vi "processCamera.vi"(0 "S arrays":T2, 1 "index":i32, 3 "B [T]":dbl=1.0, 5 "Clibration":T7={"cam 0"={"incident ANGLE COMPENSATION"=[], "field of view /pixel"=0.0, "dp/B [MeV/C/B]"=[], "charge compensation"=[], "Momentum [MeV/C]"=[], "B [T]"=1.0, "energyDependence Input"=[], "pixel angle (y)"=[], "dp [MeV/C/] "=[], "angle 2Dfor spectrumj"=[], "dp [MeV/C] 2D"=[], "charge compensation 2D"=[], "Screen&Camera 2"={"Screen Orientation"="Regular", "Screen angle"="Flat", "Lens"=enum."FL1-f8x08", "Calibration (mm/pix)"=1.0}, "ROI info"={"npix-X"=0, "npix-Y"=0, "Left [pix]"=0.0, "Top [pix]"=0.0}, "Y 2D full angle"=[]}, "cam 1"={"incident ANGLE COMPENSATION"=[], "field of view /pixel"=0.0, "dp/B [MeV/C/B]"=[], "charge compensation"=[], "Momentum [MeV/C]"=[], "B [T]"=1.0, "energyDependence Input"=[], "pixel angle (y)"=[], "dp [MeV/C/] "=[], "angle 2Dfor spectrumj"=[], "dp [MeV/C] 2D"=[], "charge compensation 2D"=[], "Screen&Camera 2"={"Screen Orientation"="Regular", "Screen angle"="Flat", "Lens"=enum."FL1-f8x08", "Calibration (mm/pix)"=1.0}, "ROI info"={"npix-X"=0, "npix-Y"=0, "Left [pix]"=0.0, "Top [pix]"=0.0}, "Y 2D full angle"=[]}, "cam 2"={"incident ANGLE COMPENSATION"=[], "field of view /pixel"=0.0, "dp/B [MeV/C/B]"=[], "charge compensation"=[], "Momentum [MeV/C]"=[], "B [T]"=1.0, "energyDependence Input"=[], "pixel angle (y)"=[], "dp [MeV/C/] "=[], "angle 2Dfor spectrumj"=[], "dp [MeV/C] 2D"=[], "charge compensation 2D"=[], "Screen&Camera 2"={"Screen Orientation"="Regular", "Screen angle"="Flat", "Lens"=enum."FL1-f8x08", "Calibration (mm/pix)"=1.0}, "ROI info"={"npix-X"=0, "npix-Y"=0, "Left [pix]"=0.0, "Top [pix]"=0.0}, "Y 2D full angle"=[]}, "cam 3"={"incident ANGLE COMPENSATION"=[], "field of view /pixel"=0.0, "dp/B [MeV/C/B]"=[], "charge compensation"=[], "Momentum [MeV/C]"=[], "B [T]"=1.0, "energyDependence Input"=[], "pixel angle (y)"=[], "dp [MeV/C/] "=[], "angle 2Dfor spectrumj"=[], "dp [MeV/C] 2D"=[], "charge compensation 2D"=[], "Screen&Camera 2"={"Screen Orientation"="Regular", "Screen angle"="Flat", "Lens"=enum."FL1-f8x08", "Calibration (mm/pix)"=1.0}, "ROI info"={"npix-X"=0, "npix-Y"=0, "Left [pix]"=0.0, "Top [pix]"=0.0}, "Y 2D full angle"=[]}}, 9 "CamSettings":T3={"Cam 0"={"position"=0.0, "Field of view"=0.0, "start"=0.0, "end"=0.0, "center"=0.0, "Lens"=enum."FL1-f8x08", "Forward"=enum."off", "Spec_Calib_file 2"=path "Y:/100TWdata/ESMCalib/datFwd.txt", "map"=path "Y:/100TWdata/ESMCalib/mapFwd.txt", "y size"=0}, "Cam 1"={"position"=0.0, "Field of view"=0.0, "start"=0.0, "end"=0.0, "center"=0.0, "Lens"=enum."FL1-f8x08", "Forward"=enum."off", "Spec_Calib_file 2"=path "Y:/100TWdata/ESMCalib/datFwd.txt", "map"=path "Y:/100TWdata/ESMCalib/mapFwd.txt", "y size"=0}, "Cam 2"={"position"=0.0, "Field of view"=0.0, "start"=0.0, "end"=0.0, "center"=0.0, "Lens"=enum."FL1-f8x08", "Forward"=enum."off", "Spec_Calib_file 2"=path "Y:/100TWdata/ESMCalib/datFwd.txt", "map"=path "Y:/100TWdata/ESMCalib/mapFwd.txt", "y size"=0}, "Cam 3"={"position"=0.0, "Field of view"=0.0, "start"=0.0, "end"=0.0, "center"=0.0, "Lens"=enum."FL1-f8x08", "Forward"=enum."off", "Spec_Calib_file 2"=path "Y:/100TWdata/ESMCalib/datFwd.txt", "map"=path "Y:/100TWdata/ESMCalib/mapFwd.txt", "y size"=0}}, 11 "error in (no error)":errorcluster, 12 "image in":T1, 14 "bg in":T1) -> (4 "z":dbl[][](graph), 6 "spec cluster":cluster{"dp [MeV/C]":dbl[], dbl[]}(graph), 8 "time: AllProc":u32, 10 "Cam Cluster out 2":T8={"incident ANGLE COMPENSATION"=[], "field of view /pixel"=0.0, "dp/B [MeV/C/B]"=[], "charge compensation"=[], "Momentum [MeV/C]"=[], "B [T]"=1.0, "energyDependence Input"=[], "pixel angle (y)"=[], "dp [MeV/C/] "=[], "angle 2Dfor spectrumj"=[], "dp [MeV/C] 2D"=[], "charge compensation 2D"=[], "Screen&Camera 2"={"Screen Orientation"="Regular", "Screen angle"="Flat", "Lens"=enum."FL1-f8x08", "Calibration (mm/pix)"=1.0}, "ROI info"={"npix-X"=0, "npix-Y"=0, "Left [pix]"=0.0, "Top [pix]"=0.0}, "Y 2D full angle"=[]}, 13 "Sum Y":cluster{"Ramp Pattern":dbl[], dbl[]}, 15 "error out":errorcluster)   [LabVIEW 2011, in "MagAnalysis_Online.lvclass"]
uses:
  MagAnalysis_Online.lvclass
  calib_Sub_Typdef.ctl
  ScreenCam2_TypDEf.ctl
  CamAndObj_TypDEf.ctl
  ROIInfo_TypDef.ctl
  Calib_Typdef.ctl
  CamSettings_Typdef.ctl
  CamSettingSUB_TypDEf.ctl
  OnOffTypeDef.ctl
  IMAQ Image.ctl
panel:
  out "time: cluster":u32
  out "time: process image":u32
  out "time:BG+Screws":u32
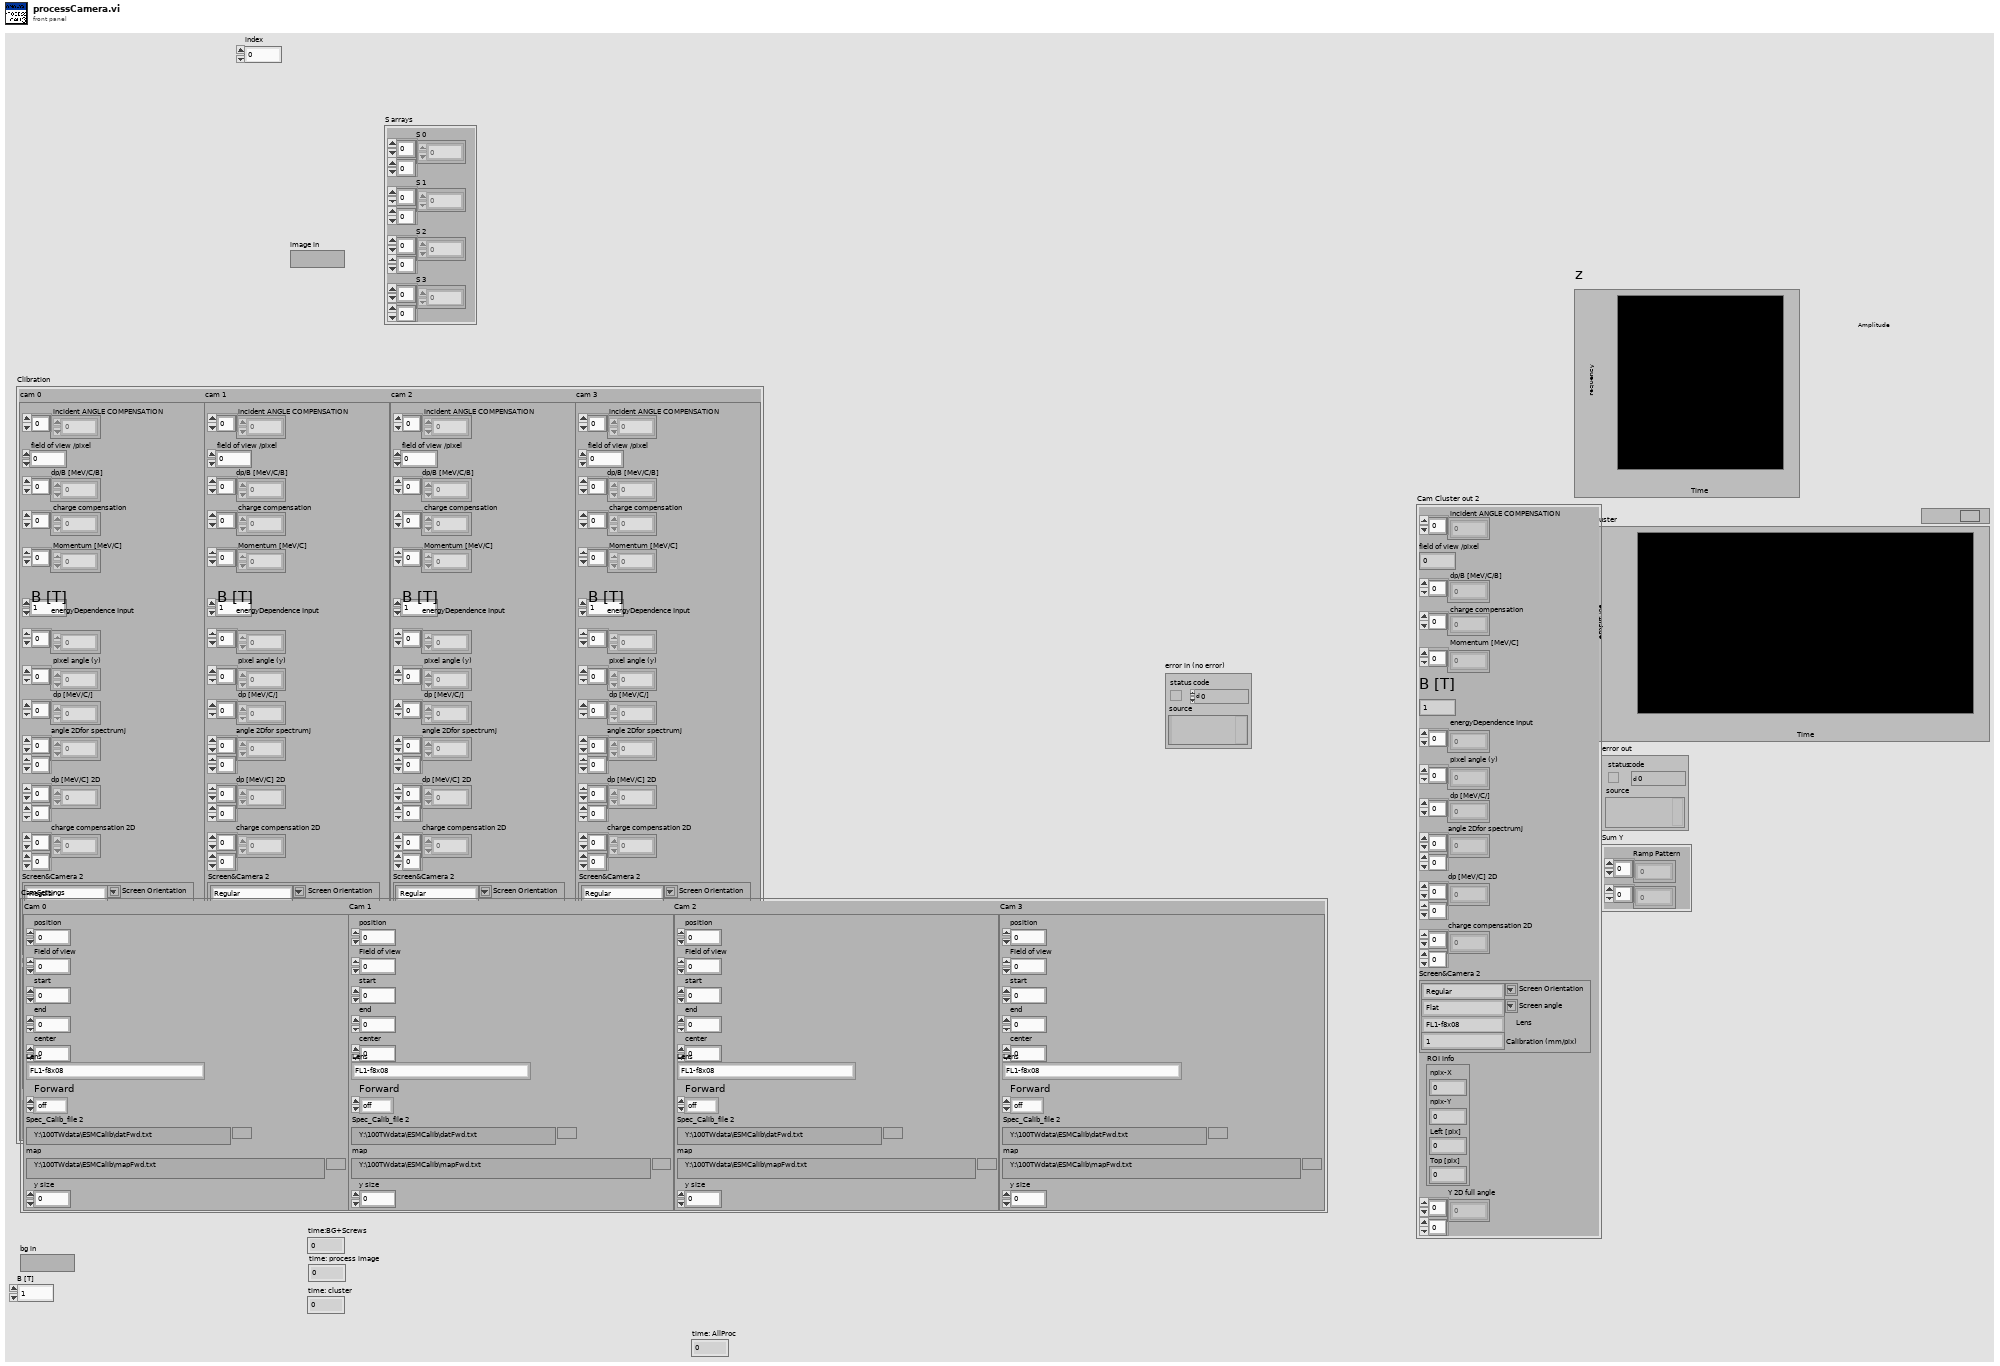
[diagram p1: front panel]
types:
  T1 = typedef "IMAQ Image.ctl" = refnum<image>
  T2 = cluster{"S 0":i32[][], "S 1":i32[][], "S 2":i32[][], "S 3":i32[][]}
  T3 = typedef "CamSettings_Typdef.ctl" = cluster{"Cam 0":T4, "Cam 1":T4, "Cam 2":T4, "Cam 3":T4}
  T4 = typedef "CamSettingSUB_TypDEf.ctl" = cluster{"position":dbl, "Field of view":dbl, "start":dbl, "end":dbl, "center":dbl, "Lens":T5, "Forward":T6, "Spec_Calib_file 2":path, "map":path, "y size":i32}
  T5 = typedef "CamAndObj_TypDEf.ctl" = enum16{"FL1-f8x08", "FL1-f8x06", "FL1-f8", "ch300-f50", "FL2G-f8", "FL3M14-f8", "FL3M14-f8x08", "FL3M14-f8x08(2x2)"}
  T6 = typedef "OnOffTypeDef.ctl" = enum16{"off", "on"}
  T7 = typedef "Calib_Typdef.ctl" = cluster{"cam 0":T8, "cam 1":T8, "cam 2":T8, "cam 3":T8}
  T8 = typedef "calib_Sub_Typdef.ctl" = cluster{"incident ANGLE COMPENSATION":dbl[], "field of view /pixel":dbl, "dp/B [MeV/C/B]":dbl[], "charge compensation":dbl[], "Momentum [MeV/C]":dbl[], "B [T]":dbl, "energyDependence Input":dbl[], "pixel angle (y)":dbl[], "dp [MeV/C/] ":dbl[], "angle 2Dfor spectrumj":dbl[][], "dp [MeV/C] 2D":dbl[][], "charge compensation 2D":dbl[][], "Screen&Camera 2":T9, "ROI info":T10, "Y 2D full angle":dbl[][]}
  T9 = typedef "ScreenCam2_TypDEf.ctl" = cluster{"Screen Orientation":string, "Screen angle":string, "Lens":T5, "Calibration (mm/pix)":dbl}
  T10 = typedef "ROIInfo_TypDef.ctl" = cluster{"npix-X":i32, "npix-Y":i32, "Left [pix]":dbl, "Top [pix]":dbl}
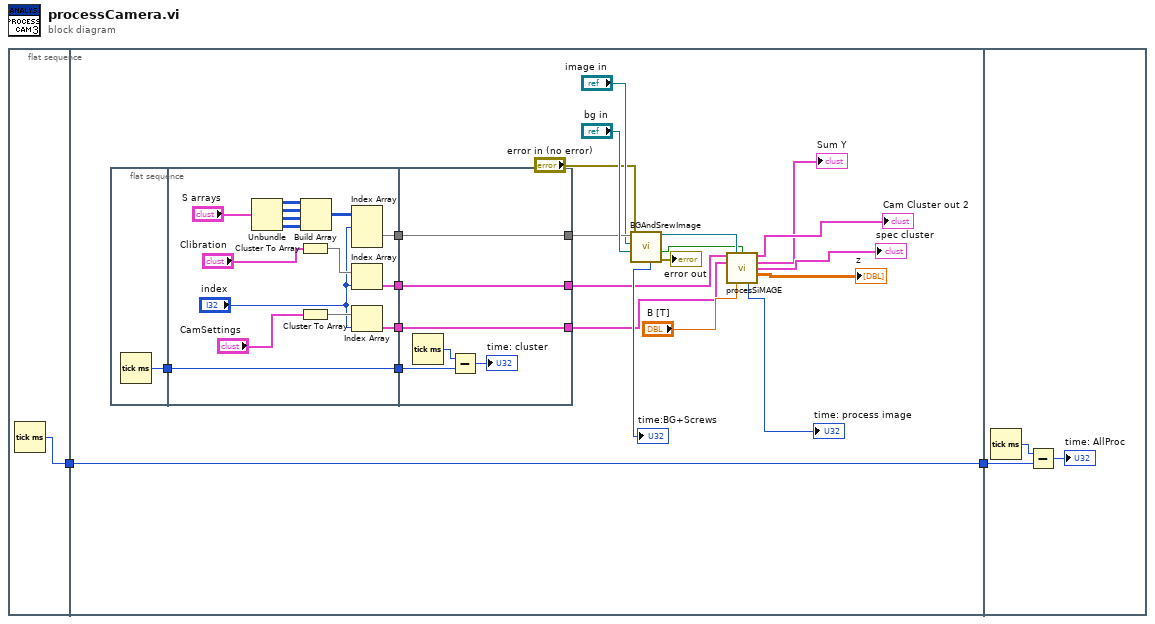
[diagram p0: block diagram]
diagram:
  n1 = flat-sequence {
    tunnel: [w3] -> w1
    tunnel: [w12] -> w2
    tunnel: w1 -> [w12]
    tunnel: w2 -> [w48]
    frame #0 {
      n2 = Tick Count (ms)() -> (millisecond timer value=w3:u32)
    }
    frame #1 {
      n3 = flat-sequence {
        tunnel: [w26] -> w25
        tunnel: [w38] -> w24
        tunnel: [w35] -> w23
        tunnel: [w27] -> w22
        tunnel: w25 -> [w41]
        tunnel: [w41] -> w21
        tunnel: [w45] -> w15
        tunnel: [w46] -> w13
        tunnel: [w47] -> w14
        tunnel: w24 -> [w47]
        tunnel: w23 -> [w46]
        tunnel: w22 -> [w45]
        tunnel: w21 -> [w42]
        frame #0 {
          n4 = Tick Count (ms)() -> (millisecond timer value=w26:u32)
        }
        frame #1 {
          n5 = Unbundle("S arrays") -> ("S 0"=w33:i32[][], "S 1"=w32:i32[][], "S 2"=w31:i32[][], "S 3"=w30:i32[][])
          n6 = Cluster To Array(cluster="Clibration") -> (array=w39:T8[])
          n7 = Cluster To Array(cluster="CamSettings") -> (array=w37:T4[])
          n8 = Build Array(w33, w32, w31, w30) -> (w29:i32[][][])
          n9 = Index Array(array=w29, index (dim 0)="index") -> (element=w27:i32[][])  [unwired: 2 in]
          n10 = Index Array(array=w39, index="index") -> (element=w38:T8)
          n11 = Index Array(array=w37, index="index") -> (element=w35:T4)
        }
        frame #2 {
          n12 = Tick Count (ms)() -> (millisecond timer value=w43:u32)
          n13 = Subtract(x=w43, y=w42) -> (x-y=→"time: cluster":u32)
        }
      }
      n14 = call "BGAndSrewImage.vi"("error in (no error)"="error in (no error)", "BG Image"="bg in", "Image"="image in", "S arrays.S 0"=w15) -> ("error out"=→"error out":errorcluster, "empty image"=w4:bool, "Image Out"=w8:T1, "time 2"=→"time:BG+Screws":u32)  [unwired: 4 in]
      n15 = call "procesSiMAGE.vi"("Cam Cluster out"=w14, "Image"=w8, "empty image"=w4, "CamSettings.Cam 0"=w13, "B [T]"="B [T]") -> ("Cam Cluster out 2"=→"Cam Cluster out 2":T8, "Sum Y"=→"Sum Y":cluster{"Ramp Pattern":dbl[], dbl[]}, "spec cluster"=→"spec cluster":cluster{"dp [MeV/C]":dbl[], dbl[]}, "z"=→"z":dbl[][], "time"=→"time: process image":u32)  [unwired: 6 in]
    }
    frame #2 {
      n16 = Tick Count (ms)() -> (millisecond timer value=w50:u32)
      n17 = Subtract(x=w50, y=w48) -> (x-y=→"time: AllProc":u32)
    }
  }
